vi "paths_2_enum.vi"(2 "file-paths":path[](array[path])) -> (6 "enum-data":cluster{"String":string, "Value":string}[](array[cluster]))   [LabVIEW 2014]
doc: "Andre Koelewijn, 6 may 2017\n\nThis VI converts an array with paths to an array with enum data for a system-type enum"
uses:
  <vilib>/Utility/miscctls.llb/LVComboBoxStrsAndValuesArrayTypeDef.ctl
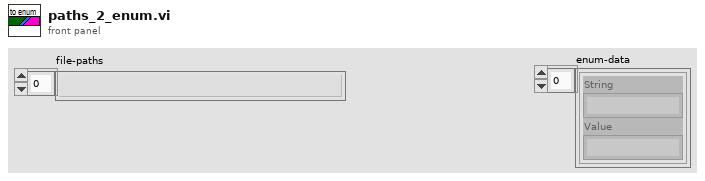
[diagram p1: front panel]
types:
  T1 = typedef "LVComboBoxStrsAndValuesArrayTypeDef.ctl" = cluster{"String":string, "Value":string}[]
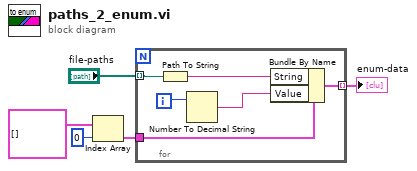
[diagram p0: block diagram]
diagram:
  n1 = Index Array(array=T1 [] ("Strings And Values []"), index=0) -> (element=w3:cluster{"String":string, "Value":string})
  n2 = for {
    tunnel: "file-paths" -> [w11] mode=indexing
    tunnel: w3 -> [w10]
    tunnel: [w6] -> w1 mode=indexing
    i -> [w8]
    n3 = Path To String(path=w11) -> (string=w9:string)
    n4 = Number To Decimal String(number=w8) -> (decimal integer string=w7:string)  [unwired: 1 in]
    n5 = Bundle By Name(cluster=w10, "String"=w9, "Value"=w7) -> (w6:cluster{"String":string, "Value":string})
  }
  "enum-data" <- w1
